vi "Demo - Generate a Sine Wave.vi"(8 "Vertical Offset":i16, 9 "Peak Amplitude":i16, 10 "Phase Offset (Radians)":dbl, 11 "Number of Samples":i32) -> (3 "Sine Wave":i16[](array[numeric]))   [LabVIEW 2017]
doc: "Generates a single sine wave, with a phase offset."
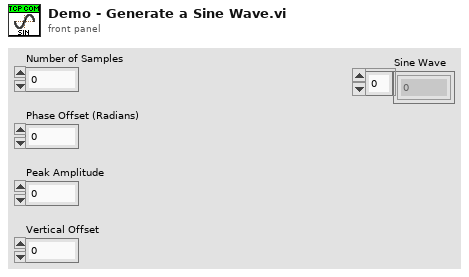
[diagram p1: front panel]
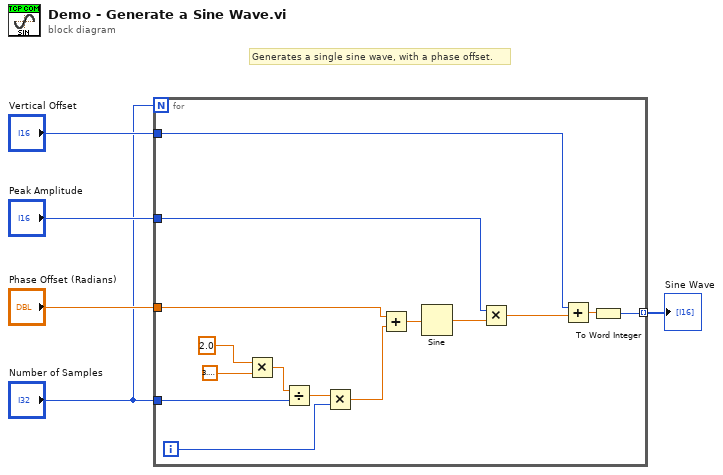
[diagram p0: block diagram]
diagram:
  # "Generates a single sine wave, with a phase offset."
  n1 = for {
    N: "Number of Samples" -> [_]
    tunnel: "Vertical Offset" -> [w20]
    tunnel: "Peak Amplitude" -> [w19]
    tunnel: "Phase Offset (Radians)" -> [w17]
    tunnel: "Number of Samples" -> [w15]
    tunnel: [w6] -> w1 mode=indexing
    i -> [w10]
    n2 = Multiply(x=2.0, y=3.141592653589793) -> (x*y=w14:dbl)
    n3 = Divide(x=w14, y=w15) -> (x/y=w11:dbl)
    n4 = Multiply(x=w11, y=w10) -> (x*y=w9:dbl)
    n5 = Add(x=w17, y=w9) -> (x+y=w16:dbl)
    n6 = Sine(x=w16) -> (sin(x)=w18:dbl)
    n7 = Multiply(x=w19, y=w18) -> (x*y=w8:dbl)
    n8 = Add(x=w20, y=w8) -> (x+y=w7:dbl)
    n9 = To Word Integer(number=w7) -> (16bit integer=w6:i16)
  }
  "Sine Wave" <- w1
